vi "test Import Export RAF CD.vi"(8 "error in (no error)":errorcluster, 11 "TestCase in":refnum<class "Routing and Faulting Scripting Unit Tests.lvclass">) -> (0 "error out":errorcluster, 3 "TestCase out":refnum<class "Routing and Faulting Scripting Unit Tests.lvclass">)   [LabVIEW 2020, in "Routing and Faulting Scripting Unit Tests.lvclass"]
uses:
  Routing and Faulting Scripting Unit Tests.lvclass
  Shared/Channel States.ctl
  Shared/Routing State.ctl
  Shared/Connection.ctl
  Routing and Faulting Scripting Unit Tests.lvclass/Routing and Faulting Scripting Unit Tests.ctl
  <userlib>/_OpenG.lib/file/file.llb/Append Path to Root if Relative - Scalar__ogtk.vi
  <vilib>/addons/_JKI Toolkits/VI Tester/TestCase.llb/TestCase.lvclass
  Routing and Faulting Scripting.lvlib
  Shared/Routing and Faulting Shared.lvlib
  niveristand-custom-device-testing-tools/VeriStandTestUtilities/VeriStandTestUtilities.lvlib
  C:/Program Files (x86)/National Instruments/LabVIEW 2020/vi.lib/addons/_JKI Toolkits/VI Tester/TestCase.llb/TestCase.lvclass
panel:
  in  "Save?":bool
  out "Output Filename":string
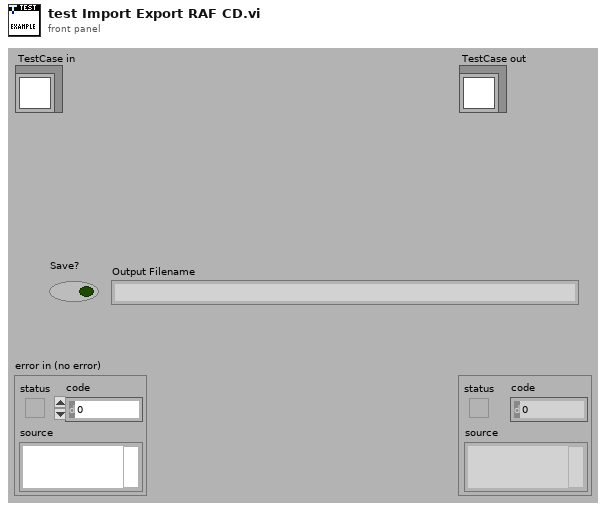
[diagram p1: front panel]
types:
  T1 = enum16{"open", "replace", "create", "open or create", "replace or create", "replace or create with confirmation"}
  T2 = typedef "Routing and Faulting Shared.lvlib/Channel States.ctl" = T3[]
  T3 = typedef "Routing and Faulting Shared.lvlib/Routing State.ctl" = cluster{"Name":string, "Description":string, "Value":i32, "Connection List":T4[]}
  T4 = typedef "Routing and Faulting Shared.lvlib/Connection.ctl" = cluster{"Module":string, "Source":string, "Destination":string}
  T5 = typedef "Custom Device API.lvlib/Custom Device Item Ref.ctl" = u64
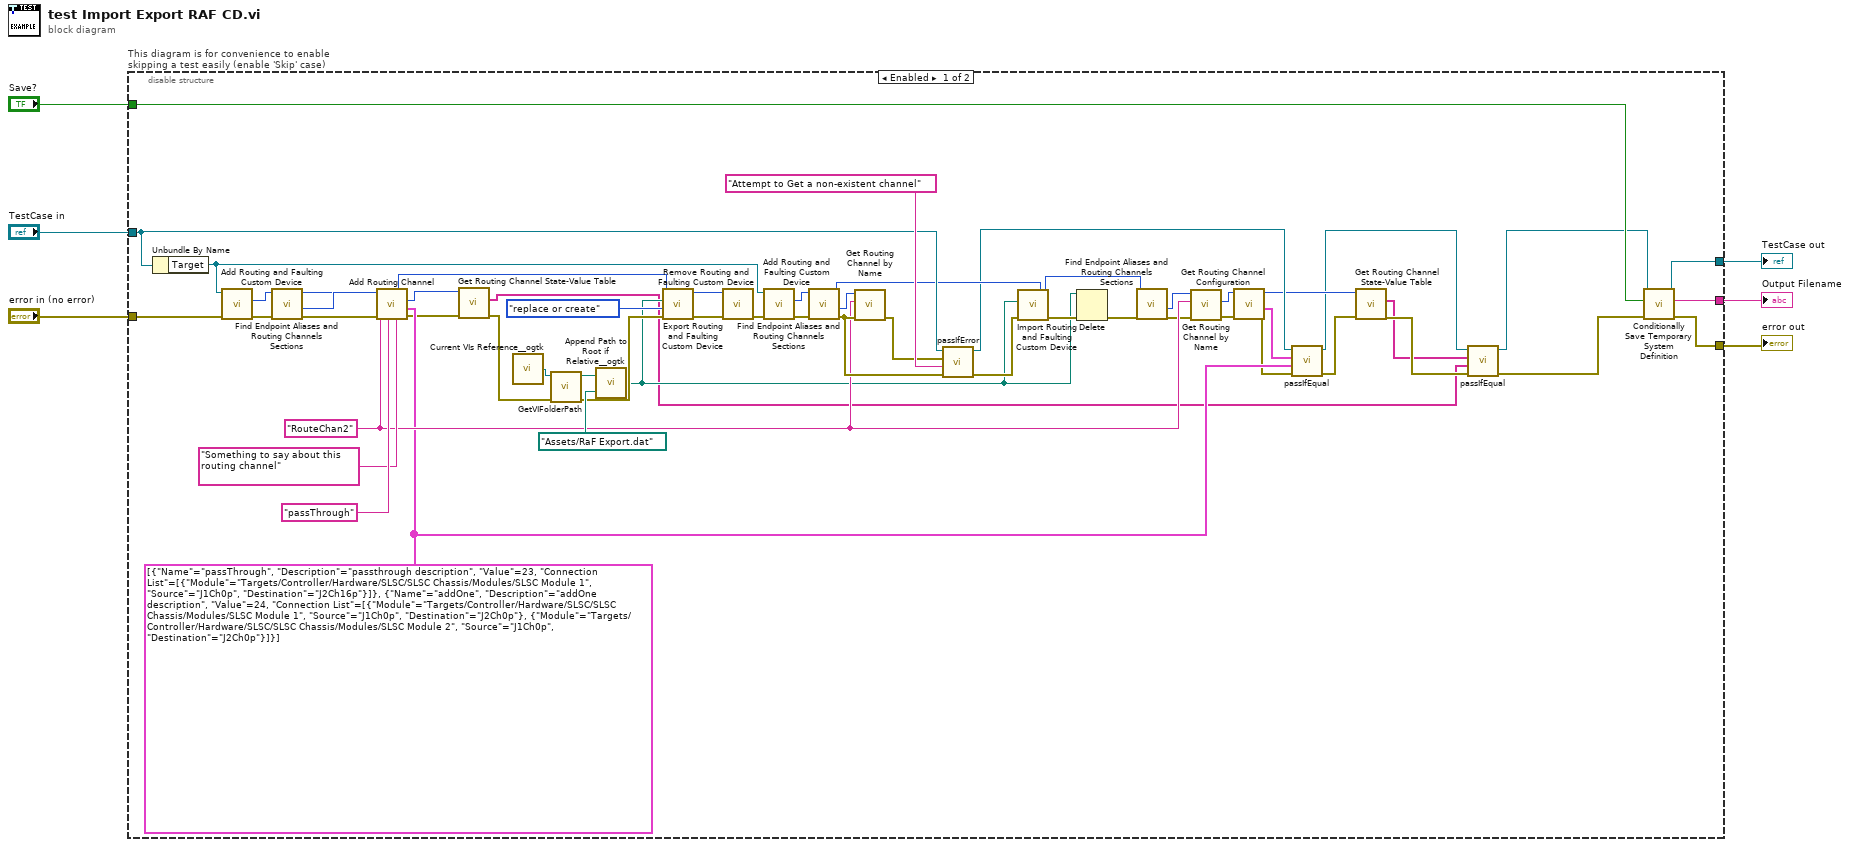
[diagram p0: block diagram]
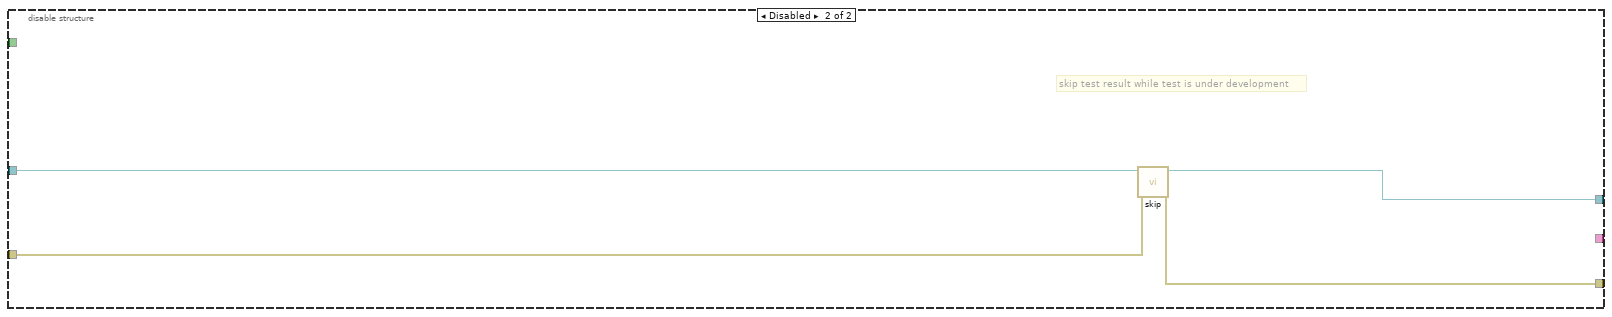
[diagram p2: hidden frame]
diagram:
  n1 = disable-structure "This diagram is for convenience to enable skipping a test easily (enable 'Skip' case)" shown="Enabled" {
    disable-tunnel: "TestCase in" -> [w41 w64]
    disable-tunnel: [w56 w62] -> w3
    disable-tunnel: [w59 w63] -> w5
    disable-tunnel: "error in (no error)" -> [w60 w61]
    disable-tunnel: [w58 _] -> w2
    disable-tunnel: "Save?" -> [w57 _]
    frame Enabled {
      w23 = T2 [{"Name"="passThrough", "Description"="passthrough description", "Value"=23, "Connection List"=[{"Module"="Targets/Controller/Hardware/SLSC/SLSC Chassis/Modules/SLSC Module 1", "Source"="J1Ch0p", "Destination"="J2Ch16p"}]}, {"Name"="addOne", "Description"="addOne description", "Value"=24, "Connection List"=[{"Module"="Targets/Controller/Hardware/SLSC/SLSC Chassis/Modules/SLSC Module 1", "Source"="J1Ch0p", "Destination"="J2Ch0p"}, {"Module"="Targets/Controller/Hardware/SLSC/SLSC Chassis/Modules/SLSC Module 2", "Source"="J1Ch0p", "Destination"="J2Ch0p"}]}] ("Channel States")
      w29 = "RouteChan2" ("Channel Name")
      n2 = Unbundle By Name(w41) -> ("Target"=w39:refnum<k24>)
      n3 = call "Add Routing and Faulting Custom Device.vi"("error in"=w60, "target in"=w39) -> ("error out"=w55:errorcluster, "routing and faulting custom device"=w54:T5)  [unwired: 7 in, 1 out]
      n4 = call "Find Endpoint Aliases and Routing Channels Sections.vi"("error in"=w55, "routing and faulting custom device in"=w54) -> ("error out"=w51:errorcluster, "routing channels"=w52:T5, "routing and faulting custom device out"=w47:T5)  [unwired: 6 in, 1 out]
      n5 = call "Add Routing Channel.vi"("description"="Something to say about this routing channel" ("Description"), "initial state"="passThrough" ("Name"), "error in"=w51, "state configurations"=w23, "channel name"=w29, "routing channels in"=w52) -> ("error out"=w16:errorcluster, "routing channel"=w15:T5)  [unwired: 3 in, 1 out]
      n6 = call "Get Routing Channel State-Value Table.vi"("error in"=w16, "routing channel in"=w15) -> ("error out"=w17:errorcluster, "state names"=w10:string[])  [unwired: 6 in, 2 out]
      n7 = call <userlib>:"Current VIs Reference__ogtk.vi"() -> ("Current VI's reference"=w50:refnum<vi>)  [unwired: 5 in]
      n8 = call "GetVIFolderPath.vi"("error in (no error)"=w17, "VI Reference in"=w50) -> ("error out"=w46:errorcluster, "VI Folder Path out"=w49:path)  [unwired: 8 in]
      n9 = call-poly <userlib>:"Append Path to Root if Relative__ogtk.vi"("Absolute or Relative Path"=path "Assets/RaF Export.dat", "Root Path"=w49) -> ("Absolute or Appended Path"=w18:path)
      n10 = call "Export Routing and Faulting Custom Device.vi"("error in"=w46, "operation"=T1."replace or create", "datalog path (use dialog)"=w18, "routing and faulting custom device in"=w47) -> ("error out"=w43:errorcluster, "routing and faulting custom device out"=w44:T5)  [unwired: 6 in]
      n11 = call "Remove Routing and Faulting Custom Device.vi"("error in"=w43, "routing and faulting custom device"=w44) -> ("error out"=w38:errorcluster)  [unwired: 9 in]
      n12 = call "Add Routing and Faulting Custom Device.vi"("error in"=w38, "target in"=w39) -> ("error out"=w37:errorcluster, "routing and faulting custom device"=w36:T5)  [unwired: 7 in, 1 out]
      n13 = call "Find Endpoint Aliases and Routing Channels Sections.vi"("error in"=w37, "routing and faulting custom device in"=w36) -> ("error out"=w33:errorcluster, "routing channels"=w35:T5, "routing and faulting custom device out"=w32:T5)  [unwired: 6 in, 1 out]
      n14 = call "Get Routing Channel by Name.vi"("error in"=w33, "channel name"=w29, "routing channels in"=w35) -> ("error out"=w34:errorcluster)  [unwired: 6 in, 2 out]
      n15 = call-dynamic "passIfError.vi"("error in (no error)"=w33, "task (\"\")"="Attempt to Get a non-existent channel" ("task (\"\")"), "error"=w34, "TestCase in"=w41) -> ("error out"=w31:errorcluster, "TestCase out"=w27:refnum<class "Routing and Faulting Scripting Unit Tests.lvclass">)  [unwired: 6 in]
      n16 = call "Import Routing and Faulting Custom Device.vi"("error in"=w31, "datalog path (use dialog)"=w18, "routing and faulting custom device in"=w32) -> ("error out"=w20:errorcluster, "routing and faulting custom device out"=w21:T5)  [unwired: 7 in]
      n17 = Delete(path (use dialog)=w18, error in=w20) -> (error out=w19:errorcluster)  [unwired: 3 in, 2 out]
      n18 = call "Find Endpoint Aliases and Routing Channels Sections.vi"("error in"=w19, "routing and faulting custom device in"=w21) -> ("error out"=w28:errorcluster, "routing channels"=w30:T5)  [unwired: 6 in, 2 out]
      n19 = call "Get Routing Channel by Name.vi"("error in"=w28, "channel name"=w29, "routing channels in"=w30) -> ("error out"=w25:errorcluster, "routing channel"=w26:T5)  [unwired: 6 in, 1 out]
      n20 = call "Get Routing Channel Configuration.vi"("error in"=w25, "routing channel in"=w26) -> ("error out"=w22:errorcluster, "state configurations"=w24:T2, "routing channel out"=w14:T5)  [unwired: 4 in, 3 out]
      n21 = call-dynamic "passIfEqual.vi"("error in (no error)"=w22, "y"=w23, "x"=w24, "TestCase in"=w27) -> ("error out"=w13:errorcluster, "TestCase out"=w8:refnum<class "Routing and Faulting Scripting Unit Tests.lvclass">)  [unwired: 6 in]
      n22 = call "Get Routing Channel State-Value Table.vi"("error in"=w13, "routing channel in"=w14) -> ("error out"=w12:errorcluster, "state names"=w11:string[])  [unwired: 6 in, 2 out]
      n23 = call-dynamic "passIfEqual.vi"("error in (no error)"=w12, "y"=w10, "x"=w11, "TestCase in"=w8) -> ("error out"=w9:errorcluster, "TestCase out"=w7:refnum<class "Routing and Faulting Scripting Unit Tests.lvclass">)  [unwired: 6 in]
      n24 = call "Conditionally Save Temporary System Definition.vi"("error in (no error)"=w9, "Save?"=w57, "Test Case"=w7) -> ("error out"=w59:errorcluster, "filename"=w58:string, "Test Case"=w56:refnum<class "Routing and Faulting Scripting Unit Tests.lvclass">)  [unwired: 6 in]
    }
    frame Disabled {
      # "skip test result while test is under development"
      n25 = call <vilib>:"skip.vi"("error in (no error)"=w61, "TestCase in"=w64) -> ("error out"=w63:errorcluster, "TestCase out"=w62:refnum<class "Routing and Faulting Scripting Unit Tests.lvclass">)  [unwired: 8 in]
    }
  }
  "error out" <- w5
  "TestCase out" <- w3
  "Output Filename" <- w2
